vi "RS232 Simulation.vi"(11 "Message Queues out":T1) -> ()   [LabVIEW 2024]
doc: "This VI Used to simulate the reading from RS 232"
uses:
  Message Queue/All Message Queues.ctl
  Message Queue/Message Cluster.ctl
  controls/GlobalData.ctl
  <userlib>/_OpenG.lib/numeric/numeric.llb/Random Number Within Range - DBL__ogtk.vi
  <vilib>/Instr/_visa.llb/VISA Configure Serial Port (Instr).vi
  Message Queue/Enqueue Message (Single).vi
  controls/GlobalData.vi
  <userlib>/_OpenG.lib/numeric/numeric.llb/openg_numeric__ogtk.lvlib
  Message Queue/Message Queue.lvlib
panel:
  out "error out 2":errorcluster
  out "error out":errorcluster
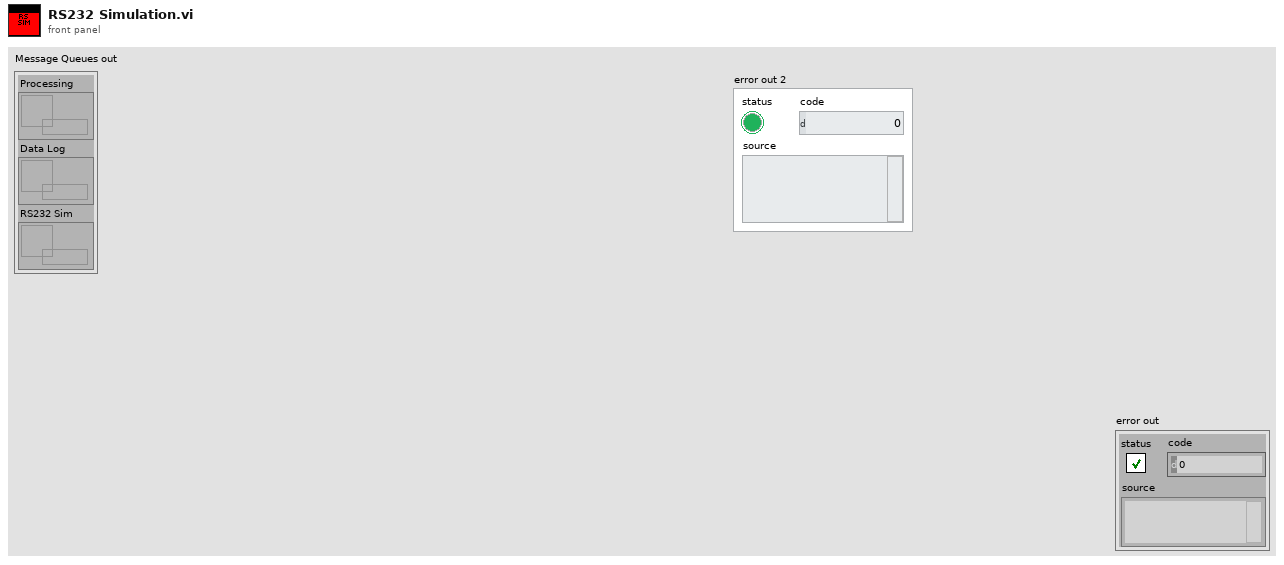
[diagram p1: front panel]
types:
  T1 = typedef "Message Queue.lvlib/All Message Queues.ctl" = cluster{"Processing":refnum<queue>, "Data Log":refnum<queue>, "RS232 Sim":refnum<queue>}
  T2 = typedef "GlobalData.ctl" = cluster{"Measurements":cluster{"Measurement Graphs":refnum<vi>, "Pressure":refnum<vi>, "Temperature":refnum<vi>, "Salinity":refnum<vi>, "Weight":refnum<vi>, "Pressure Raw":refnum<vi>, "Temperature Raw":refnum<vi>, "Salinity Raw":refnum<vi>, "Weight Raw":refnum<vi>, "Measurement Statstics":refnum<vi>, "Time Array":refnum<vi>}, "Settings":cluster{"Sampling Settings":refnum<vi>, "General Settings":refnum<vi>, "Disable Sensor Reading":refnum<vi>, "Units Settings":refnum<vi>, "Channels Settings":refnum<vi>, "Weight Port Settings":refnum<vi>}, "Calibration Data":cluster{"Pressure Cal":refnum<vi>, "Temperature Cal":refnum<vi>, "Salinity Cal":refnum<vi>, "Weight Cal":refnum<vi>}, "UI":cluster{"Generate Report":refnum<vi>}}
  T3 = typedef "Serial - Settings.ctl" = cluster{"baud rate":u32, "data bits":u16, "parity":enum16{"None", "Odd", "Even", "Mark", "Space"}, "stop bits":u16, "flow control":u16}
  T4 = cluster{"Port Name":refnum<visa-resource-name>, "Port Settings":T3}
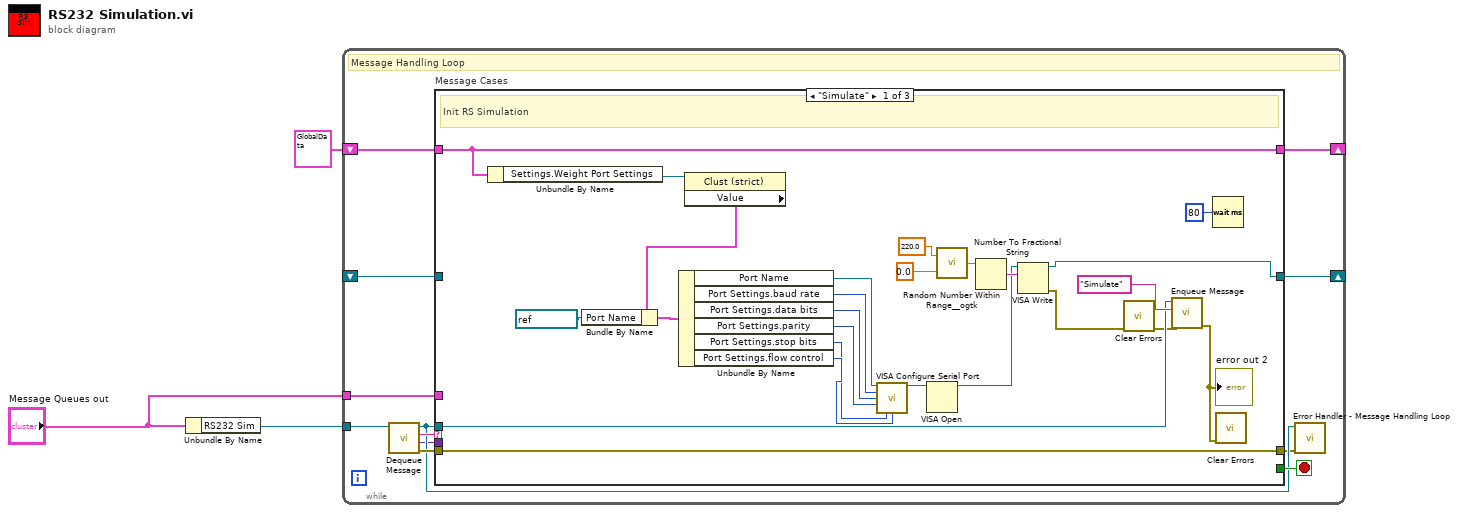
[diagram p0: block diagram]
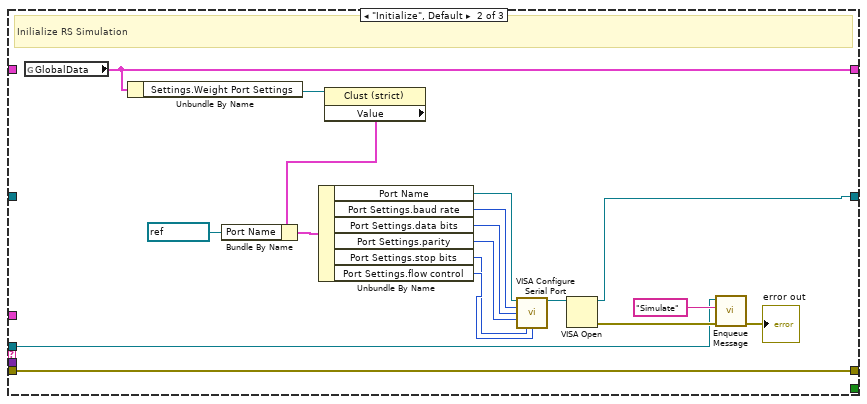
[diagram p2: hidden frame]
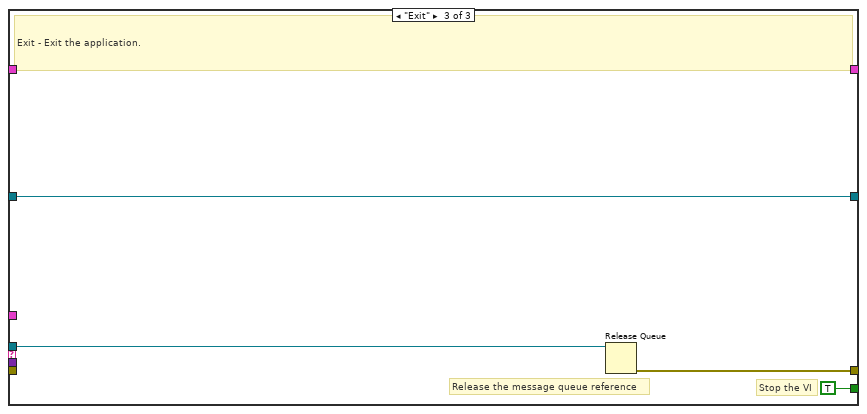
[diagram p3: hidden frame]
diagram:
  n1 = Unbundle By Name("Message Queues out") -> ("RS232 Sim"=w3:refnum<queue>)
  n2 = while {
    tunnel: w3 -> [w10]
    shift-right: [w14] -> _
    shift-left: T2 {"Measurements"={"Measurement Graphs"=refnum, "Pressure"=refnum, "Temperature"=refnum, "Salinity"=refnum, "Weight"=refnum, "Pressure Raw"=refnum, "Temperature Raw"=refnum, "Salinity Raw"=refnum, "Weight Raw"=refnum, "Measurement Statstics"=refnum, "Time Array"=refnum}, "Settings"={"Sampling Settings"=refnum, "General Settings"=refnum, "Disable Sensor Reading"=refnum, "Units Settings"=refnum, "Channels Settings"=refnum, "Weight Port Settings"=refnum}, "Calibration Data"={"Pressure Cal"=refnum, "Temperature Cal"=refnum, "Salinity Cal"=refnum, "Weight Cal"=refnum}, "UI"={"Generate Report"=refnum}} ("GlobalData") -> [w15]
    shift-right: [w6] -> _
    shift-left: _ -> [w5]
    tunnel: "Message Queues out" -> [w4]
    stop <- w13 stop-if-true
    # "Message Handling Loop"
    n3 = call "Dequeue Message.vi"("Message Queue"=w10) -> ("error out"=w12:errorcluster, "Message Data"=w7:variant, "Message"=w11:string, "dup Message Queue"=w9:refnum<queue>)  [unwired: 7 in]
    n4 = case "Message Cases" shown="\"Simulate\"" w11 {
      tunnel: w9 -> [w35 w42 w63]
      tunnel: w12 -> [w33 w41 _]
      tunnel: [w33 w41 w59] -> w8
      tunnel: w15 -> [w17 _ w62]
      tunnel: [w17 w57 w62] -> w14
      tunnel: [_ _ TRUE] -> w13
      tunnel: w7 -> [_ _ _]
      tunnel: [w34 w58 w60] -> w6
      tunnel: w5 -> [_ _ w60]
      tunnel: w4 -> [_ _ _]
      frame "Simulate" {
        # "Init RS Simulation"
        n5 = Unbundle By Name(w17) -> ("Settings.Weight Port Settings"=w28:refnum<vi>)
        n6 = property class="Clust (strict)"(reference=w28) -> ("Value"=w27:T4)  [unwired: 1 in, 2 out]
        n7 = Bundle By Name(cluster=w27, "Port Name"=refnum<visa-resource-name> "COM1") -> (w19:T4)
        n8 = Unbundle By Name(w19) -> ("Port Name"=w26:refnum<visa-resource-name>, "Port Settings.baud rate"=w24:u32, "Port Settings.data bits"=w23:u16, "Port Settings.parity"=w22:enum16{"None", "Odd", "Even", "Mark", "Space"}, "Port Settings.stop bits"=w21:u16, "Port Settings.flow control"=w25:u16)
        n9 = call-poly "VISA Configure Serial Port"("VISA resource name"=w26, "baud rate (9600)"=w24, "data bits (8)"=w23, "parity (0:none)"=w22, "stop bits (10: 1 bit)"=w21, "flow control (0:none)"=w25) -> ("VISA resource name out"=w20:refnum<visa-resource-name>)  [unwired: 3 in, 6 out]
        n10 = VISA Open(VISA resource name=w20) -> (VISA resource name=w16:refnum<visa-resource-name>)  [unwired: 4 in, 1 out]
        n11 = call-poly <userlib>:"Random Number Within Range__ogtk.vi"("High"=220.0, "Low"=0.0) -> ("Random Number"=w39:dbl)  [unwired: 3 in]
        n12 = Number To Fractional String(number=w39) -> (F-format string=w40:string)  [unwired: 3 in]
        n13 = VISA Write(VISA resource name=w16, write buffer=w40) -> (VISA resource name out=w34:refnum<visa-resource-name>, error out=w31:errorcluster)  [unwired: 1 in, 1 out]
        n14 = call <vilib>:"Clear Errors.vi"("error in (no error)"=w31) -> ("error out"=w30:errorcluster)  [unwired: 5 in, 1 out]
        n15 = call-poly "Enqueue Message.vi"("error in (no error)"=w30, "Message"="Simulate", "Message Queue"=w35) -> ("error out"=w32:errorcluster)  [unwired: 7 in, 1 out]
        "error out 2" <- w32
        n16 = Wait (ms)(milliseconds to wait=u32 80) -> ()  [unwired: 1 out]
        n17 = call <vilib>:"Clear Errors.vi"("error in (no error)"=w32) -> ()  [unwired: 5 in, 2 out]
      }
      frame "Initialize", Default {
        # "Inilialize RS Simulation"
        n18 = global read "GlobalData.vi" "GlobalData"() -> (w57:T2)
        n19 = Unbundle By Name(w57) -> ("Settings.Weight Port Settings"=w56:refnum<vi>)
        n20 = property class="Clust (strict)"(reference=w56) -> ("Value"=w55:T4)  [unwired: 1 in, 2 out]
        n21 = Bundle By Name(cluster=w55, "Port Name"=refnum<visa-resource-name> "COM1") -> (w44:T4)
        n22 = Unbundle By Name(w44) -> ("Port Name"=w54:refnum<visa-resource-name>, "Port Settings.baud rate"=w52:u32, "Port Settings.data bits"=w51:u16, "Port Settings.parity"=w50:enum16{"None", "Odd", "Even", "Mark", "Space"}, "Port Settings.stop bits"=w49:u16, "Port Settings.flow control"=w53:u16)
        n23 = call-poly "VISA Configure Serial Port"("VISA resource name"=w54, "baud rate (9600)"=w52, "data bits (8)"=w51, "parity (0:none)"=w50, "stop bits (10: 1 bit)"=w49, "flow control (0:none)"=w53) -> ("VISA resource name out"=w48:refnum<visa-resource-name>)  [unwired: 3 in, 6 out]
        n24 = VISA Open(VISA resource name=w48) -> (VISA resource name=w58:refnum<visa-resource-name>, error out=w46:errorcluster)  [unwired: 4 in]
        n25 = call-poly "Enqueue Message.vi"("error in (no error)"=w46, "Message"="Simulate", "Message Queue"=w42) -> ("error out"=→"error out":errorcluster)  [unwired: 7 in, 1 out]
      }
      frame "Exit" {
        # "Stop the VI"
        # "Release the message queue reference"
        # "Exit - Exit the application."
        n26 = Release Queue(queue=w63) -> (error out=w59:errorcluster)  [unwired: 2 in, 2 out]
      }
    }
    n27 = call "Error Handler - Message Handling Loop.vi"("error in (no error)"=w8, "Message Queue"=w9) -> ()  [unwired: 8 in, 2 out]
  }
